vi "GetPerspectiveTransform.vi"(8 "error in":errorcluster, 9 "DecompTypes":T1 items=["DECOMP_LU"=0, "DECOMP_SVD"=1, "DECOMP_EIG"=2, "DECOMP_CHOLESKY"=3, "DECOMP_QR"=4, "DECOMP_NORMAL"=16], 10 "Dst":T2[](array[typedef]), 11 "Src":T2[](array[typedef])) -> (0 "error out":errorcluster, 3 "Result":dbl[][](array[numeric]))   [LabVIEW 2020, in "OpenLvVision_OpenCv.lvlib"]
doc: "Calculates a perspective transform from four pairs of the corresponding points."
uses:
  OpenLvVision_OpenCv.lvlib
  TypeDef/Point/2D_PointSGL.ctl
  TypeDef/DecompTypes.ctl
  Dlls/OlvOpenCvWrapper.dll
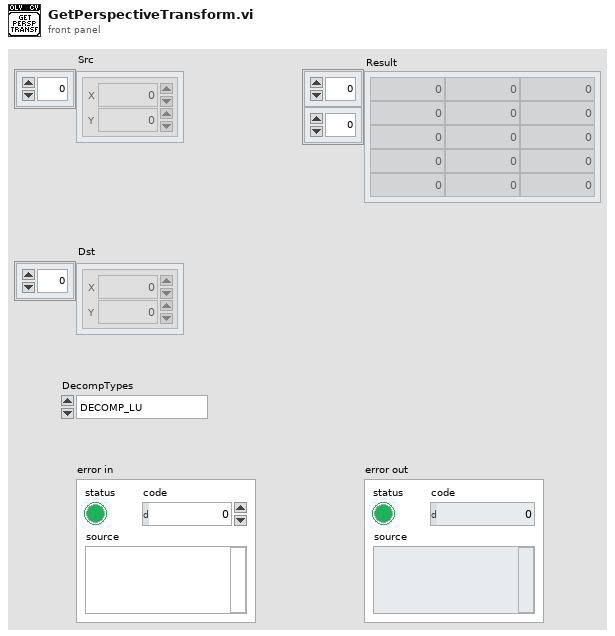
[diagram p1: front panel]
types:
  T1 = typedef "OpenLvVision_OpenCv.lvlib/DecompTypes.ctl" = i32
  T2 = typedef "OpenLvVision_OpenCv.lvlib/2D_PointSGL.ctl" = cluster{"X":sgl, "Y":sgl}
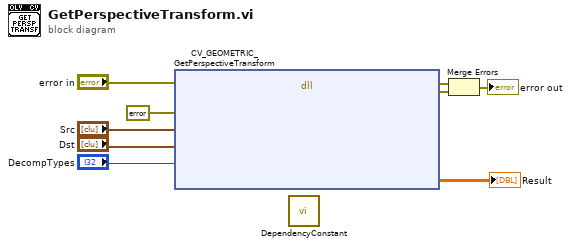
[diagram p0: block diagram]
diagram:
  n1 = dll-call lib="C:/Users/lukas/Downloads/OpenLvVision_OpenCv/SourceCode/LabView/OpenLvVision_OpenCv/Dlls/OlvOpenCvWrapper.dll" fn="CV_GEOMETRIC_GetPerspectiveTransform"(error in="error in", "Error"=errorcluster {"status"=FALSE, "code"=0, "source"=""}, "src"="Src", "dst"="Dst", "solveMethod"="DecompTypes") -> (error out=w7:errorcluster, "Error"=w8:errorcluster, "result"=→"Result":dbl[][])  [unwired: 7 in, 1 out]
  n2 = call "DependencyConstant.vi"() -> ()  [unwired: 12 in]
  n3 = Merge Errors(w7, w8) -> (→"error out":errorcluster)
